vi "16- SLOPE VI.vi"() -> ()   [LabVIEW 2018]
panel:
  in  "stop":bool
  out "Numeric":dbl
  in  "X1":dbl
  in  "X2":dbl
  in  "Y1":dbl
  in  "Y2":dbl
  # "WAP to display the slope of a line"
  # "(y2-y1)+(x2-x1)=m"
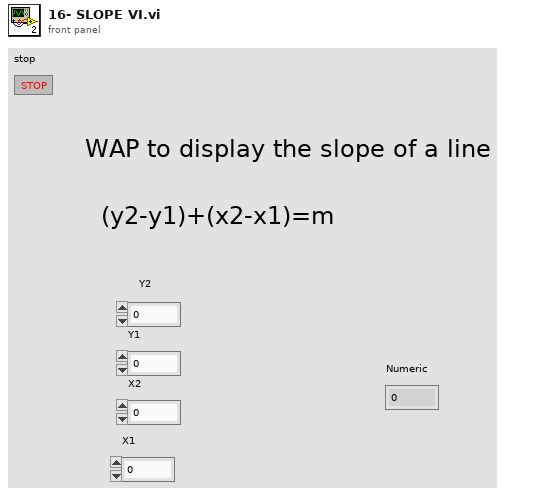
[diagram p1: front panel]
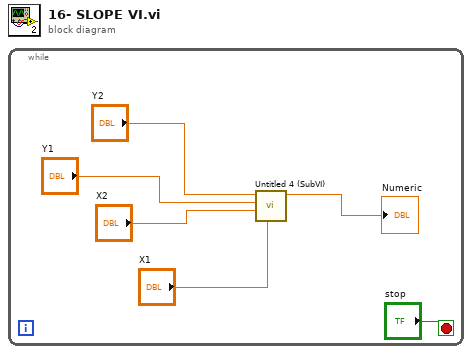
[diagram p0: block diagram]
diagram:
  n1 = while {
    stop <- "stop" stop-if-true
    n2 = call "Untitled 4 (SubVI).vi"("X1"="X1", "X2"="X2", "Y1"="Y1", "Y2"="Y2") -> ("Numeric"=→"Numeric":dbl)  [unwired: 7 in]
  }
